vi "Set Trigger Mode.vi"(8 "error in (no error)":errorcluster, 11 "Trigger Mode?":bool) -> (0 "error out":errorcluster)   [LabVIEW 2013]
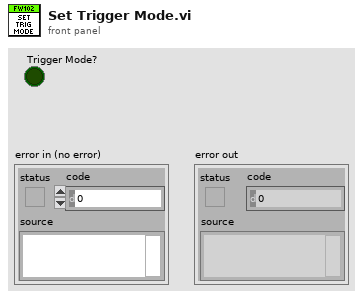
[diagram p1: front panel]
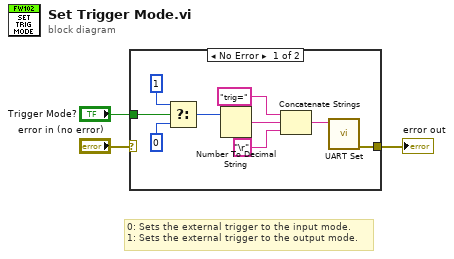
[diagram p0: block diagram]
diagram:
  # "0: Sets the external trigger to the input mode.\n1: Sets the external trigger to the output mode."
  n1 = case shown="No Error" "error in (no error)" {
    selector: "error in (no error)" -> [_ w13]
    tunnel: [w12 w13] -> w3
    tunnel: "Trigger Mode?" -> [w11 _]
    frame No Error {
      n2 = Select(t=1, s=w11, f=0) -> (s? t:f=w4:i32)
      n3 = Number To Decimal String(number=w4) -> (decimal integer string=w10:string)  [unwired: 1 in]
      n4 = Concatenate Strings("trig=" ("Input Command String"), w10, "\r" ("string")) -> (w7:string)
      n5 = call "UART Set.vi"("Command"=w7) -> ("error out"=w12:errorcluster)  [unwired: 10 in]
    }
    frame Error {
    }
  }
  "error out" <- w3
